vi "Threat_Manager.vi"(8 "PIR":dbl, 9 "Freeze":bool, 10 "Seuil CRC":dbl, 11 "Nb CRC invalides":dbl) -> (3 "Threat Level":dbl)   [LabVIEW 2022 SP3]
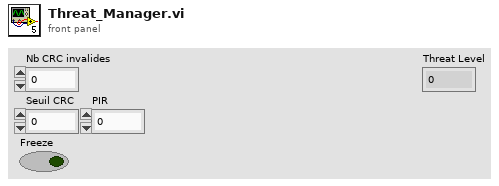
[diagram p1: front panel]
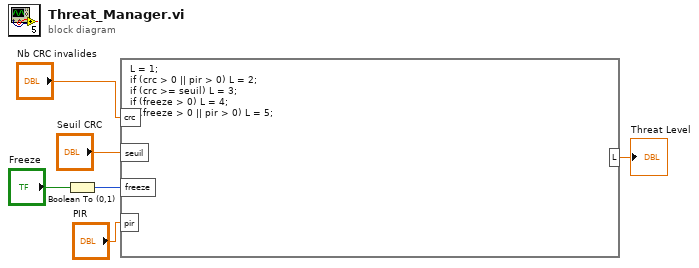
[diagram p0: block diagram]
diagram:
  n1 = Boolean To (0,1)(Boolean="Freeze") -> (0, 1=w2:i16)
  n2 = formula code="L = 1;\nif (crc > 0 || pir > 0) L = 2;\nif (crc >= seuil) L = 3;\nif (freeze > 0) L = 4;\nif (freeze > 0 || pir > 0) L = 5;"("crc"="Nb CRC invalides", "seuil"="Seuil CRC", "freeze"=w2, "pir"="PIR") -> ("L"=→"Threat Level":dbl)
